vi "Read Sequence Name.vi"(8 "error in (no error)":errorcluster, 11 "SequenceRepo in":refnum<class "SequenceRepo.lvclass">) -> (0 "error out":errorcluster, 2 "Sequence Name":string, 3 "SequenceRepo out":refnum<class "SequenceRepo.lvclass">)   [LabVIEW 2015, in "SequenceRepo.lvclass"]
uses:
  SequenceRepo.lvclass
  SequenceRepo.lvclass/SequenceRepo.ctl
  Prototype/classes/Sequence/Config/Sequence Config.lvclass
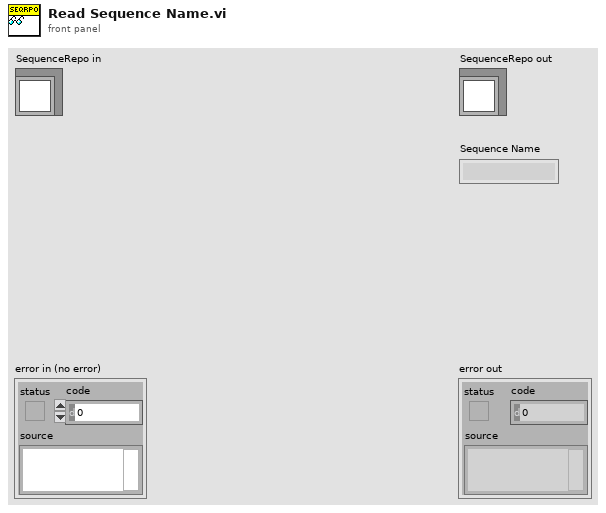
[diagram p1: front panel]
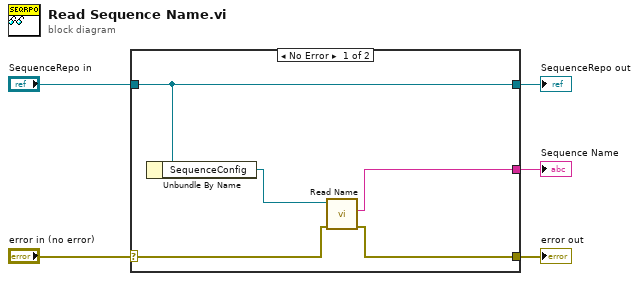
[diagram p0: block diagram]
diagram:
  n1 = case shown="No Error" "error in (no error)" {
    selector: "error in (no error)" -> [w8 w11]
    tunnel: [w7 w11] -> w4
    tunnel: [w10 w12] -> w2
    tunnel: "SequenceRepo in" -> [w10 w12]
    tunnel: [w6 _] -> w1
    frame No Error {
      n2 = Unbundle By Name(w10) -> ("SequenceConfig"=w9:refnum<class "Sequence Config.lvclass">)
      n3 = call-dynamic "Read Name.vi"("error in (no error)"=w8, "Sequence in"=w9) -> ("error out"=w7:errorcluster, "Name"=w6:string)  [unwired: 7 in, 1 out]
    }
    frame Error {
    }
  }
  "error out" <- w4
  "SequenceRepo out" <- w2
  "Sequence Name" <- w1
